vi "Add time to CSV report.vi"(10 "Time":string, 11 "SerialNumber":string) -> (0 "error out":errorcluster)   [LabVIEW 2020, in "CSV Report.lvlib"]
uses:
  CSV Report.lvlib
panel:
  out "concatenated string":string
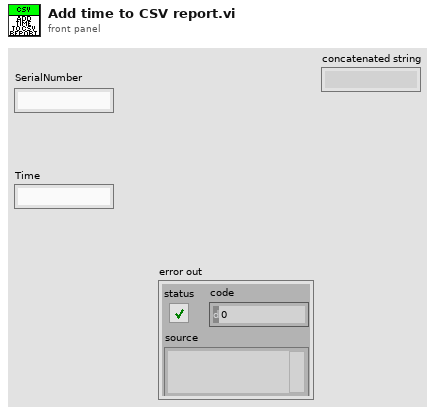
[diagram p1: front panel]
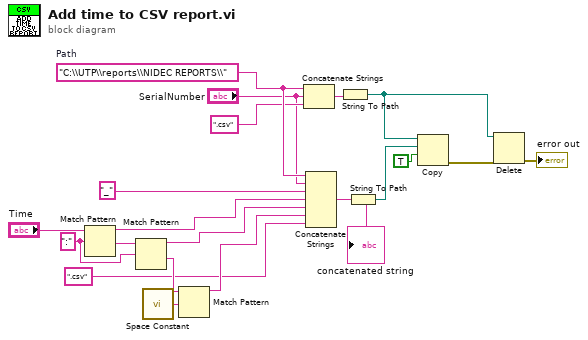
[diagram p0: block diagram]
diagram:
  w15 = "C:\\UTP\\reports\\NIDEC REPORTS\\"  # Path
  w19 = ":" ("regular expression")
  n1 = Match Pattern(string="Time", regular expression=w19) -> (before substring=w12:string, after substring=w20:string)  [unwired: 1 in, 2 out]
  n2 = Match Pattern(string=w20, regular expression=w19) -> (before substring=w11:string, after substring=w18:string)  [unwired: 1 in, 2 out]
  n3 = call <vilib>:"Space Constant.vi"() -> ("String"=w17:string)
  n4 = Match Pattern(string=w18, regular expression=w17) -> (before substring=w10:string)  [unwired: 1 in, 3 out]
  n5 = Concatenate Strings(w15, "SerialNumber", ".csv") -> (w16:string)
  n6 = Concatenate Strings(w15, "SerialNumber", "_" ("string"), w12, w11, w10, ".csv" ("string")) -> (w7:string)
  "concatenated string" <- w7
  n7 = String To Path(string=w16) -> (path=w3:path)
  n8 = String To Path(string=w7) -> (path=w6:path)
  n9 = Copy(9:TRUE ("overwrite (F)"), 10:w6, 11:w3) -> (0:w4:errorcluster)  [unwired: 2 in, 2 out]
  n10 = Delete(path (use dialog)=w3, error in=w4) -> (error out=→"error out":errorcluster)  [unwired: 3 in, 2 out]
